vi "add_string.vi"   [LabVIEW 2016]
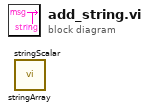
[diagram p0: block diagram]
diagram:
  n1 = call "stringArray.vi"() -> ()  [unwired: 5 in, 1 out]
  n2 = call "stringScalar.vi"() -> ()  [unwired: 5 in, 1 out]
